vi "UIReadCtrl.vi"(8 "error in":errorcluster, 10 "Control Label":string, 11 "UI Ref cluster in":T1) -> (0 "error out":errorcluster, 1 "Control Value":variant, 2 "Found":bool, 3 "UI Ref cluster out":T1, 5 "CtrlRef":refnum<vi>)   [LabVIEW 2025, in "UI_Library.lvlib" / "UI_Library.lvclass"]
doc: "Read Control value"
uses:
  UI_Library.lvclass
  Controls/UI_RefCluster.ctl
  <vilib>/Utility/Data Type/Type Definitions/Data Type.ctl
  UI_Library.lvlib
  <vilib>/Utility/Data Type/NI_Data Type.lvlib
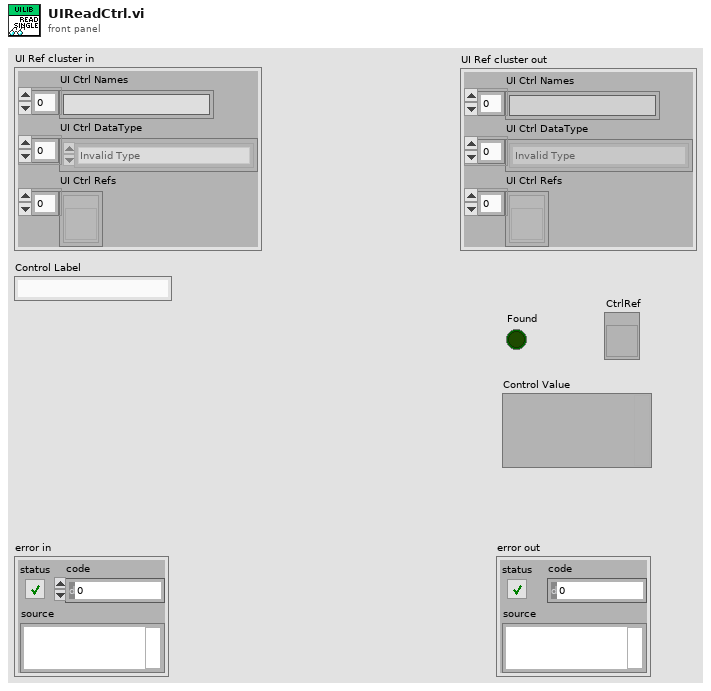
[diagram p1: front panel]
types:
  T1 = typedef "UI_Library.lvlib/UI_RefCluster.ctl" = cluster{"UI Ctrl Names":string[], "UI Ctrl DataType":T2[], "UI Ctrl Refs":refnum<vi>[]}
  T2 = typedef "NI_Data Type.lvlib/Data Type.ctl" = enum8{"Invalid Type", "Void", "I8", "I16", "I32", "I64", "U8", "U16", "U32", "U64", "Single Float", "Double Float", "Extended Float", "Single Complex", "Double Complex", "Extended Complex", "Enum U8", "Enum U16", "Enum U32", "Enum U64", "Single Float With Unit", "Double Float With Unit", "Extended Float With Unit", "Single Complex with Unit", "Double Complex with Unit", "Extended Complex with Unit", "Boolean", "String", "Path", "Picture", "Tag", "Array", "Cluster", "Variant", "LV Variant", "Waveform", "Timestamp", "Digital Waveform", "Digital Data", "ExpressData", "Refnum", "External Data", "VI", "Poly VI", "LabVIEW Class Instance", "Fixed Point", "Set Collection", "Map Collection"}
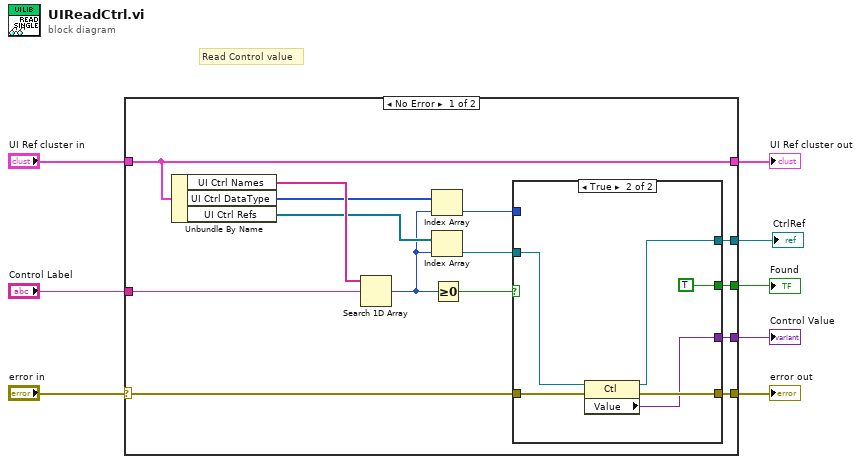
[diagram p0: block diagram]
diagram:
  # "Read Control value"
  n1 = case shown="No Error" "error in" {
    selector: "error in" -> [w14 w31]
    tunnel: [w13 w31] -> w8
    tunnel: "Control Label" -> [w21 _]
    tunnel: [w12 w30] -> w5
    tunnel: "UI Ref cluster in" -> [w12 w30]
    tunnel: [w11 _] -> w3
    tunnel: [w10 _] -> w2
    tunnel: [w9 _] -> w1
    frame No Error {
      n2 = Unbundle By Name(w12) -> ("UI Ctrl Names"=w22:string[], "UI Ctrl DataType"=w19:T2[], "UI Ctrl Refs"=w18:refnum<vi>[])
      n3 = Search 1D Array(1D array=w22, element=w21) -> (index of element=w17:i32)  [unwired: 1 in]
      n4 = Index Array(array=w19, index=w17) -> (element=w16:T2)
      n5 = Index Array(array=w18, index=w17) -> (element=w15:refnum<vi>)
      n6 = Greater Or Equal To 0?(x=w17) -> (x >= 0?=w20:bool)
      n7 = case shown="True" w20 {
        tunnel: w16 -> [_ _]
        tunnel: w15 -> [_ w28]
        tunnel: w14 -> [w23 w29]
        tunnel: [w23 w27] -> w13
        tunnel: [_ w26] -> w11
        tunnel: [_ TRUE] -> w10
        tunnel: [_ w24] -> w9
        frame False {
        }
        frame True {
          n8 = property class="Ctl"(reference=w28, error in=w29) -> (reference out=w24:refnum<vi>, error out=w27:errorcluster, "Value"=w26:variant)
        }
      }
    }
    frame Error {
    }
  }
  "error out" <- w8
  "Control Value" <- w3
  "UI Ref cluster out" <- w5
  "Found" <- w2
  "CtrlRef" <- w1
